vi "passTestResultCounter.vi"(10 "IA State":T1={"our_robots"=[], "enemy_robots"=[], "balls"=[], "geometry"={"line_width"=0, "field_length"=0, "field_width"=0, "boundary_width"=0, "referee_width"=0, "goal_width"=0, "goal_depth"=0, "goal_wall_width"=0, "center_circle_radius"=0, "defense_radius"=0, "defense_stretch"=0, "free_kick_from_defense_dist"=0, "penalty_spot_from_field_line_dist"=0, "penalty_line_from_spot_dist"=0}, "IA Judge"={"stage"="", "command"="", "our_goalie_id"=0.0, "enemy_goalie_id"=0.0, "command enum"=enum."Halt", "Time"=enum."Azul"}, "Received Timestamp"=timestamp(0 s since 1904-01-01), "Events"={"Touch"=FALSE, "Ball out"=FALSE, "id touch"=0.0, "Ball out of \nVision"=FALSE, "Ball inside \nGoalie area"=FALSE, "Robot not responding"=FALSE, "Robots responding status"=[1.0, 1.0, 1.0, 1.0, 1.0, 1.0], "Enemy Ball \nPossession"=FALSE, "Pass State"=FALSE, "id end of pass"=0.0, "Kick"=FALSE, "Id ini Possession"=0.0, "Ball Possesion"=FALSE, "Id Possesion"=0.0}}, 11 "Pass state":T10) -> (0 "Ball missed robot":string, 1 "Too much force":string, 2 "Ball out of the field":string, 3 "Pass Intercepted":string, 4 "Correct pass":string, 5 "Need more force to pass":string, 6 "Number of goals":string)   [LabVIEW 2017]
uses:
  passTestStates.ctl
  Core/AI Input.ctl
  Core/AI Robot.ctl
  Intel/Functions Enum.ctl
  Intel/AttackerStates.ctl
  Core/AI Ball.ctl
  Core/Field Size.ctl
  Core/AI Judge.ctl
  Intel/Command Enum.ctl
  Util/Events/Events.ctl
panel:
  out "Array":i16[](array[numeric])
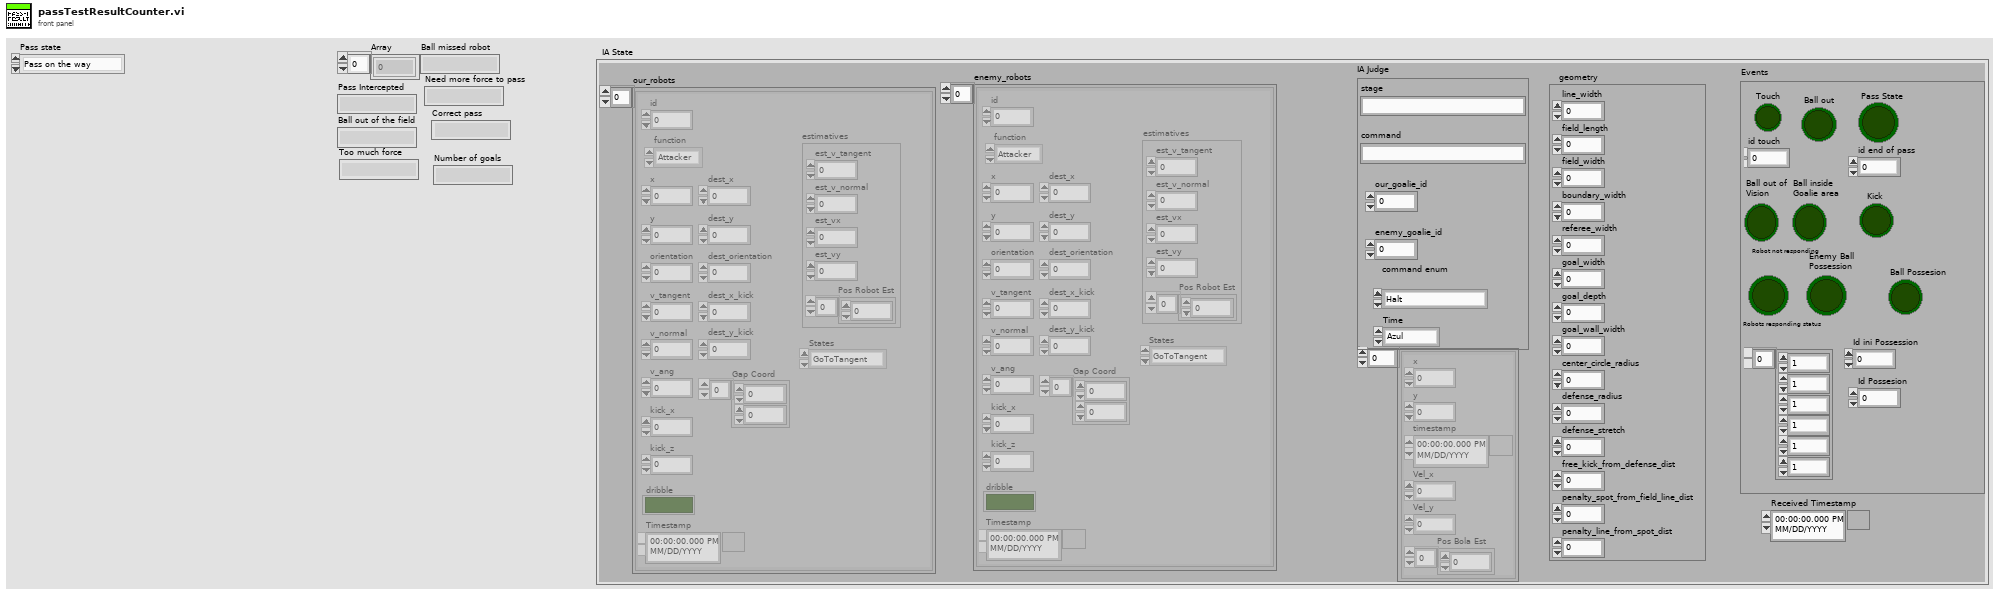
[diagram p1: front panel]
types:
  T1 = typedef "AI Input.ctl" = cluster{"our_robots":T2[], "enemy_robots":T2[], "balls":T5[], "geometry":T6, "IA Judge":T7, "Received Timestamp":timestamp, "Events":T9}
  T2 = typedef "AI Robot.ctl" = cluster{"id":u32, "function":T3, "x":dbl, "y":dbl, "orientation":dbl, "v_tangent":dbl, "v_normal":dbl, "v_ang":dbl, "kick_x":dbl, "kick_z":dbl, "dribble":bool, "Timestamp":timestamp, "dest_x":dbl, "dest_y":dbl, "dest_orientation":dbl, "estimatives":cluster{"est_v_tangent":dbl, "est_v_normal":dbl, "est_vx":dbl, "est_vy":dbl, "Pos Robot Est":dbl[]}, "dest_x_kick":dbl, "dest_y_kick":dbl, "Gap Coord":dbl[], "States":T4}
  T3 = typedef "Functions Enum.ctl" = enum16{"Attacker", "Goalie", "Defender", "Striker", "Goto 0", "Dummy", "Kicker", "ZigZag"}
  T4 = typedef "AttackerStates.ctl" = enum16{"Pass", "GoToTangent", "BallGetting", "GoToKick", ""}
  T5 = typedef "AI Ball.ctl" = cluster{"x":dbl, "y":dbl, "timestamp":timestamp, "Vel_x":dbl, "Vel_y":dbl, "Pos Bola Est":dbl[]}
  T6 = typedef "Field Size.ctl" = cluster{"line_width":u32, "field_length":u32, "field_width":u32, "boundary_width":u32, "referee_width":u32, "goal_width":u32, "goal_depth":u32, "goal_wall_width":u32, "center_circle_radius":u32, "defense_radius":u32, "defense_stretch":u32, "free_kick_from_defense_dist":u32, "penalty_spot_from_field_line_dist":u32, "penalty_line_from_spot_dist":u32}
  T7 = typedef "AI Judge.ctl" = cluster{"stage":string, "command":string, "our_goalie_id":dbl, "enemy_goalie_id":dbl, "command enum":T8, "Time":enum16{"Azul", "Amarelo"}}
  T8 = typedef "Command Enum.ctl" = enum16{"Halt", "Stop", "Force Start", "PKA Normal Start", "Prepare Kickoff Ally", "PKE Normal Start", "Prepare Kickoff Enemy", "Prepare Penalty Ally", "PPA Normal Start", "Prepare Penalty Enemy", "PPE Normal Start", "Direct Free Enemy", "Direct Free Ally", "Indirect Free Enemy", "Indirect Free Ally", "Timeout Enemy", "Timeout Ally", "Goal Enemy", "Goal Ally", "Ball Placement Enemy", "Ball Placement Ally", "Normal Half Time", "Extra Time Break", "Extra Half Time", "None", "Post Game"}
  T9 = typedef "Events.ctl" = cluster{"Touch":bool, "Ball out":bool, "id touch":dbl, "Ball out of \nVision":bool, "Ball inside \nGoalie area":bool, "Robot not responding":bool, "Robots responding status":dbl[], "Enemy Ball \nPossession":bool, "Pass State":bool, "id end of pass":dbl, "Kick":bool, "Id ini Possession":dbl, "Ball Possesion":bool, "Id Possesion":dbl}
  T10 = typedef "passTestStates.ctl" = enum16{"Pass on the way", "Ball stops", "Pass intercepted", "Ball out of the field", "Ball missed robot", "Need more force to pass", "Too much force", "Correct pass", "Keep ball possesion", "Robot kicked the ball", "Waiting Kick", "Invalid: same robot", "Invalid: kicker ID 999", "Invalid: Receiver ID 999", "Invalid"}
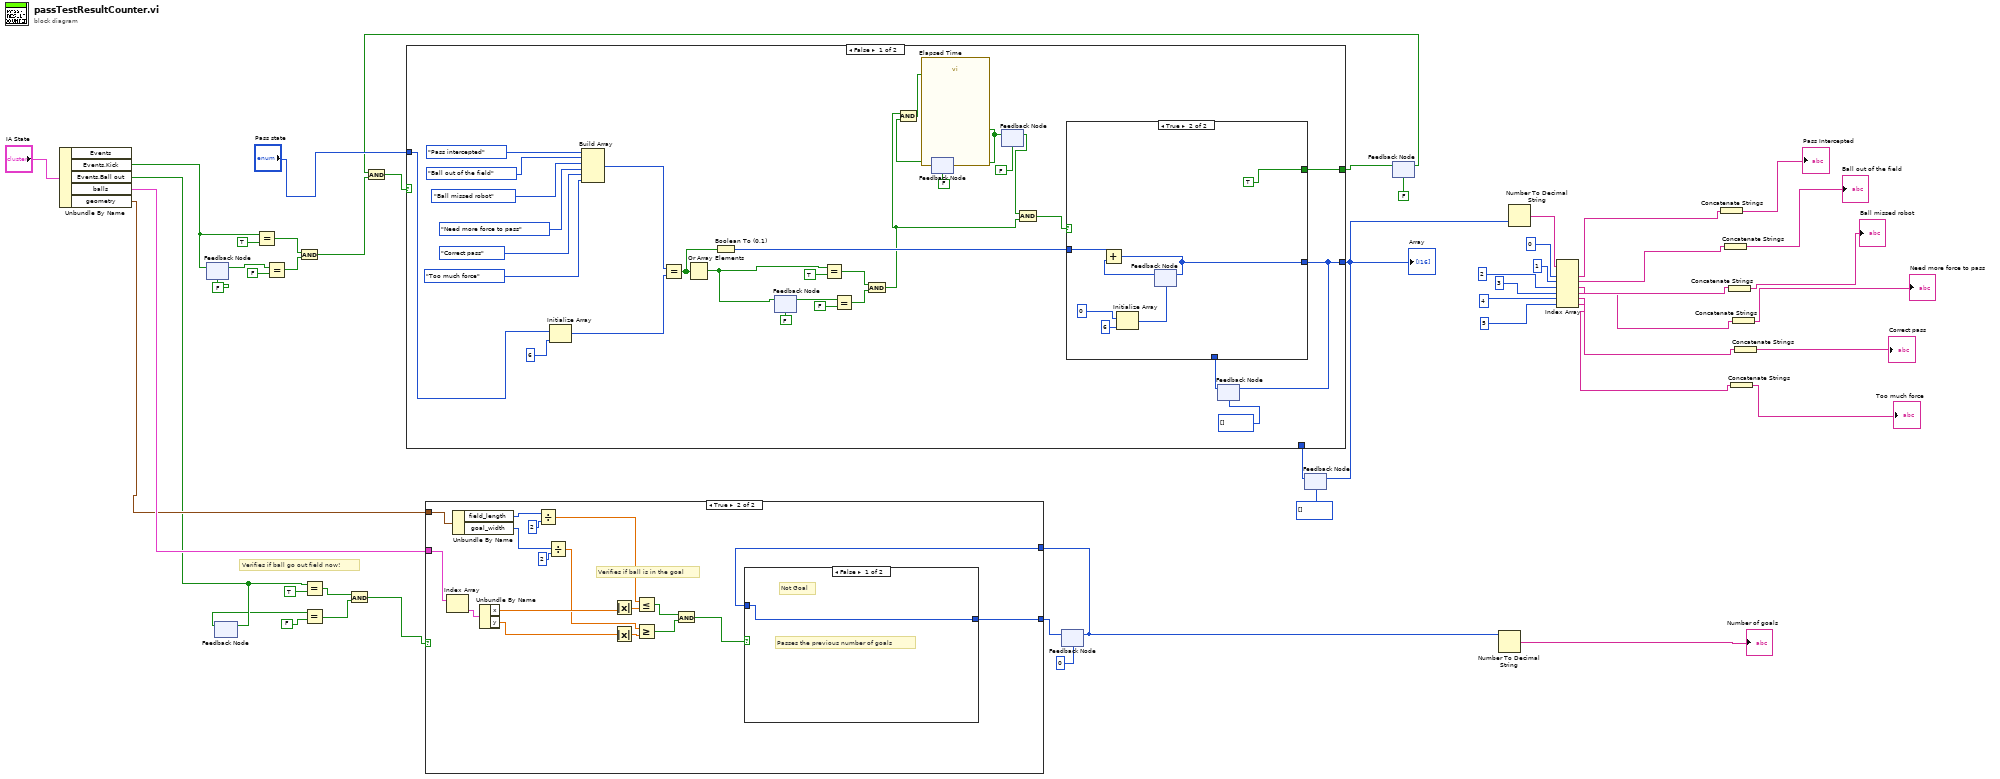
[diagram p0: block diagram]
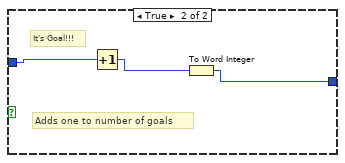
[diagram p3: hidden frame]
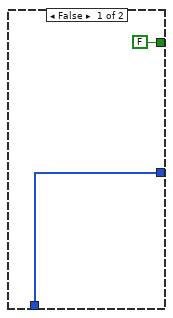
[diagram p4: hidden frame]
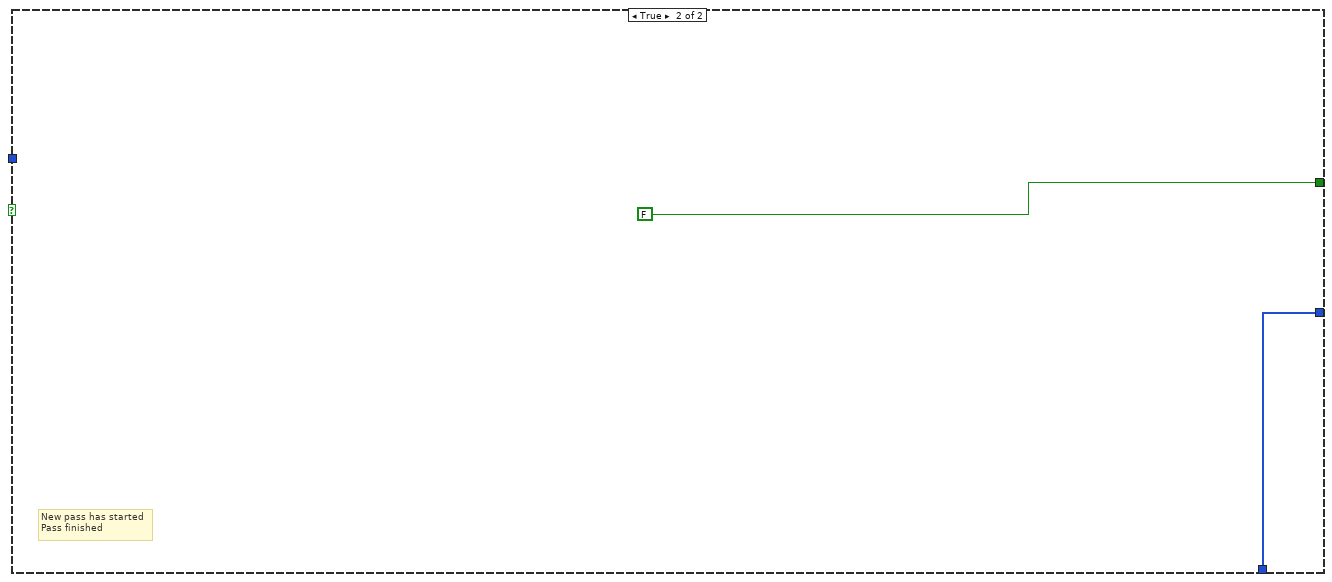
[diagram p5: hidden frame]
diagram:
  # "Verifies if ball go out field now!"
  n1 = Unbundle By Name("IA State") -> ("Events.Kick"=w41:bool, "Events.Ball out"=w2:bool, "balls"=w8:T5[], "geometry"=w7:T6)  [unwired: 1 out]
  n2 = feedback #1(FALSE ("Kick")) -> (w39:bool)
  n3 = feedback-in #1(w41) -> ()
  n4 = feedback-in #2(w2) -> ()
  n5 = feedback #2() -> (w1:bool)  [unwired: 1 in]
  n6 = Equal?(x=w41, y=TRUE) -> (x = y?=w36:bool)
  n7 = Equal?(x=w39, y=FALSE) -> (x = y?=w37:bool)
  n8 = And(x=w36, y=w37) -> (x .and. y?=w34:bool)
  n9 = Equal?(x=w2, y=TRUE) -> (x = y?=w11:bool)
  n10 = Equal?(x=w1, y=FALSE) -> (x = y?=w10:bool)
  n11 = And(x=w11, y=w10) -> (x .and. y?=w9:bool)
  n12 = feedback #3(i16 0) -> (w3:i16)
  n13 = case shown="True" w9 {
    tunnel: w8 -> [_ w68]
    tunnel: w7 -> [_ w63]
    tunnel: [w50 w52] -> w5
    tunnel: w3 -> [w50 w51]
    frame False {
      # "Passes the previous number of goals"
      # "Ball still go out field"
    }
    frame True {
      # "Verifies if ball is in the goal"
      n14 = Index Array(array=w68) -> (element=w67:T5)  [unwired: 1 in]
      n15 = Unbundle By Name(w63) -> ("field_length"=w62:u32, "goal_width"=w59:u32)
      n16 = Unbundle By Name(w67) -> ("x"=w66:dbl, "y"=w65:dbl)
      n17 = Divide(x=w62, y=u32 2) -> (x/y=w58:dbl)
      n18 = Divide(x=w59, y=u32 2) -> (x/y=w56:dbl)
      n19 = Absolute Value(x=w66) -> (abs(x)=w64:dbl)
      n20 = Absolute Value(x=w65) -> (abs(x)=w57:dbl)
      n21 = Less Or Equal?(x=w58, y=w64) -> (x <= y?=w55:bool)
      n22 = Greater Or Equal?(x=w56, y=w57) -> (x >= y?=w54:bool)
      n23 = And(x=w55, y=w54) -> (x .and. y?=w53:bool)
      n24 = case shown="False" w53 {
        tunnel: [w69 w70] -> w52
        tunnel: w51 -> [w69 w72]
        frame False {
          # "Passes the previous number of goals"
          # "Not Goal"
        }
        frame True {
          # "Adds one to number of goals"
          # "It's Goal!!!"
          n25 = Increment(x=w72) -> (x+1=w71:i16)
          n26 = To Word Integer(number=w71) -> (16bit integer=w70:i16)
        }
      }
    }
  }
  n27 = feedback-in #3(w5) -> ()
  n28 = feedback #4(i16[] [] ("0, 1")) -> (w48:i32[])
  n29 = feedback #5(FALSE) -> (w44:bool)
  n30 = And(x=w44, y=w34) -> (x .and. y?=w43:bool)
  n31 = case shown="False" w43 {
    tunnel: "Pass state" -> [w81 _]
    tunnel: [w103 FALSE] -> w46
    tunnel: [w91 w113] -> w33
    tunnel: w48 -> [_ w113]
    frame False {
      n32 = Initialize Array(w81, 6 ("dimension size")) -> (w97:T10[])
      n33 = Build Array(passTestStates."Pass intercepted" ("y"), passTestStates."Ball out of the field" ("y"), passTestStates."Ball missed robot" ("y"), passTestStates."Need more force to pass" ("y"), passTestStates."Correct pass" ("y"), passTestStates."Too much force" ("y")) -> (w95:T10[])
      n34 = Equal?(x=w95, y=w97) -> (x = y?=w94:bool[])
      n35 = Or Array Elements(Boolean array=w94) -> (logical OR=w82:bool)
      n36 = Boolean To (0,1)(Boolean=w94) -> (0, 1=w93:i16[])
      n37 = feedback #6(FALSE ("Kick")) -> (w86:bool)
      n38 = feedback-in #6(w82) -> ()
      n39 = Equal?(x=w82, y=TRUE) -> (x = y?=w83:bool)
      n40 = Equal?(x=w86, y=FALSE) -> (x = y?=w84:bool)
      n41 = And(x=w83, y=w84) -> (x .and. y?=w76:bool)
      n42 = feedback #7(FALSE ("Time has Elapsed")) -> (w77:bool)
      n43 = And(x=w76, y=w77) -> (x .and. y?=w78:bool)
      n44 = call "Elapsed Time"("Reset"=w78) -> ("Time has Elapsed"=w75:bool)  [unwired: 11 in, 7 out]
      n45 = feedback-in #7(w75) -> ()
      n46 = feedback #8(FALSE ("Time has Elapsed")) -> (w74:bool)
      n47 = feedback-in #8(w75) -> ()
      n48 = And(x=w74, y=w76) -> (x .and. y?=w80:bool)
      n49 = feedback #9(i16[] [] ("0, 1")) -> (w90:i32[])
      n50 = case shown="True" w80 {
        tunnel: [FALSE TRUE] -> w103
        tunnel: w93 -> [_ w111]
        tunnel: [w105 w109] -> w91
        tunnel: w90 -> [w105 _]
        frame False {
        }
        frame True {
          n51 = Initialize Array(0 ("dimension size"), 6 ("dimension size")) -> (w106:i32[])
          n52 = feedback #10(w106) -> (w110:i32[])
          n53 = Add(x=w111, y=w110) -> (x+y=w109:i32[])
          n54 = feedback-in #10(w109) -> ()
        }
      }
      n55 = feedback-in #9(w91) -> ()
    }
    frame True {
      # "New pass has started\nPass finished"
    }
  }
  "Array" <- w33
  n56 = feedback-in #4(w33) -> ()
  n57 = feedback-in #5(w46) -> ()
  n58 = Number To Decimal String(number=w3) -> (decimal integer string=→"Number of goals":string)  [unwired: 1 in]
  n59 = Number To Decimal String(number=w33) -> (decimal integer string=w32:string[])  [unwired: 1 in]
  n60 = Index Array(array=w32, index #1=0 ("index"), index #2=1 ("index"), index #3=2 ("index"), index #4=3 ("index"), index #5=4 ("index"), index #6=5 ("index")) -> (element #1=w31:string, element #2=w30:string, element #3=w29:string, element #4=w28:string, element #5=w27:string, element #6=w26:string)
  n61 = Concatenate Strings(w31) -> (→"Pass Intercepted":string)
  n62 = Concatenate Strings(w30) -> (→"Ball out of the field":string)
  n63 = Concatenate Strings(w29) -> (→"Ball missed robot":string)
  n64 = Concatenate Strings(w26) -> (→"Too much force":string)
  n65 = Concatenate Strings(w28) -> (→"Need more force to pass":string)
  n66 = Concatenate Strings(w27) -> (→"Correct pass":string)
